vi "TestTestJunk.vi"() -> ()   [LabVIEW 2013]
uses:
  <vilib>/regexp/Match Regular Expression.xnode
panel:
  out "String":string
  out "VP/F1 5":bool
  out "VP/F1":bool
  out "VP/F1 2":bool
  out "VP/F1 4":bool
  out "VP/F1 3":bool
  out "Pass/Fail1 2":bool
  out "Pass/Fail1":bool
  out "Pass/Fail1 4":bool
  out "Pass/Fail1 3":bool
  out "Pass/Fail1 5":bool
  out "Percent 1":dbl
  out "Percent 2":dbl
  out "Voltage 1":dbl
  out "Percent 3":dbl
  out "Percent 4":dbl
  out "Voltage 2":dbl
  out "Voltage 4":dbl
  out "Voltage 3":dbl
  out "Percent 5":dbl
  out "Voltage 5":dbl
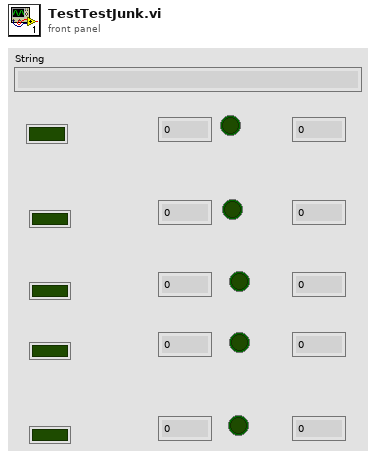
[diagram p1: front panel]
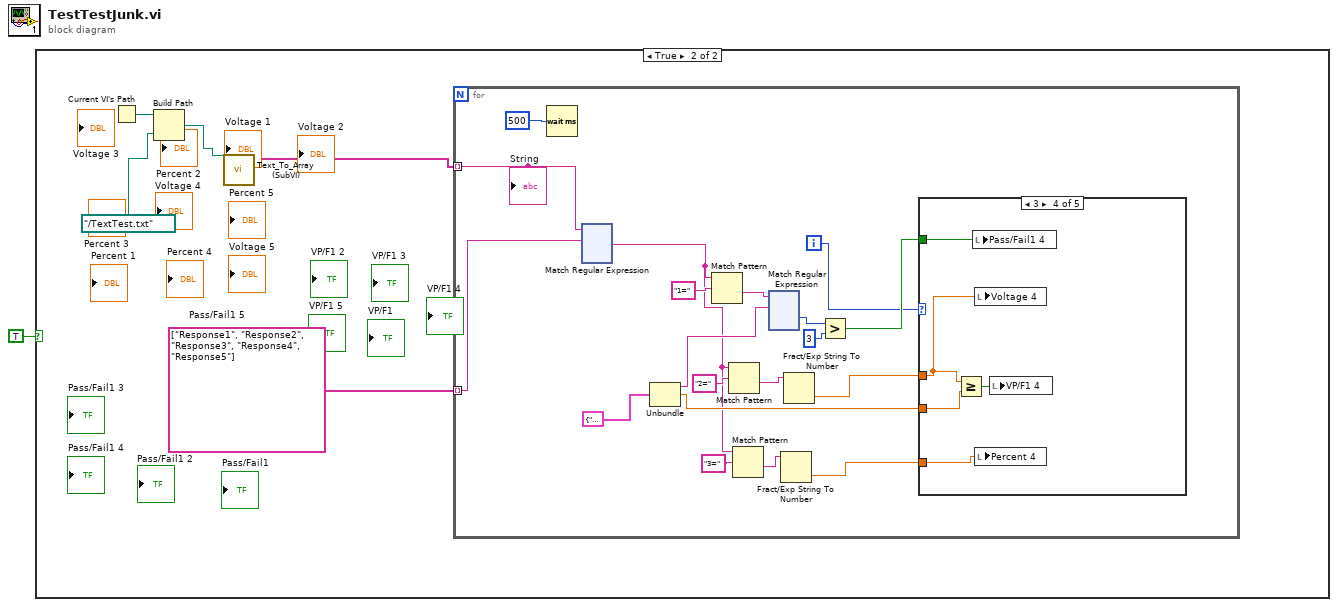
[diagram p0: block diagram]
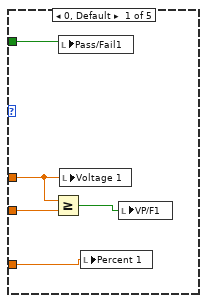
[diagram p3: hidden frame]
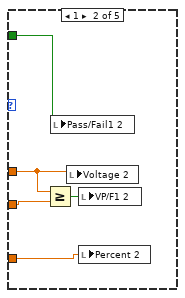
[diagram p4: hidden frame]
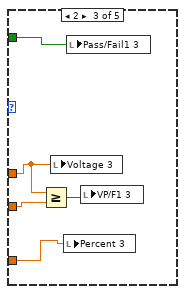
[diagram p5: hidden frame]
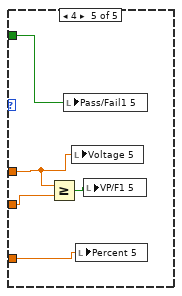
[diagram p6: hidden frame]
diagram:
  n1 = case shown="True" TRUE {
    frame False {
    }
    frame True {
      n2 = Current VI's Path() -> (path=w4:path)
      n3 = Build Path(base path=w4, name or relative path=path "../TextTest.txt") -> (appended path=w2:path)
      n4 = call "Text_To_Array (SubVI).vi"("Path"=w2) -> ("Array"=w5:string[])  [unwired: 8 in, 2 out]
      n5 = for {
        tunnel: w5 -> [w14] mode=indexing
        tunnel: string[] ["Response1", "Response2", "Response3", "Response4", "Response5"] -> [w13] mode=indexing
        i -> [w12]
        n6 = Wait (ms)(milliseconds to wait=500) -> ()  [unwired: 1 out]
        n7 = xnode "Match Regular Expression"("input string"=w14, "regular expression"=w13) -> ("after match"=w9:string)  [unwired: 4 in, 4 out]
        n8 = Unbundle(cluster{string, dbl, i32} {"PASS", 3.3, 80}) -> (w24:string, w11:dbl)  [unwired: 1 out]
        n9 = Match Pattern(string=w9, regular expression="1=") -> (after substring=w21:string)  [unwired: 1 in, 3 out]
        n10 = Match Pattern(string=w9, regular expression="2=") -> (after substring=w16:string)  [unwired: 1 in, 3 out]
        n11 = Match Pattern(string=w9, regular expression="3=") -> (after substring=w8:string)  [unwired: 1 in, 3 out]
        n12 = xnode "Match Regular Expression"("input string"=w21, "regular expression"=w24) -> ("offset past match"=w20:i32)  [unwired: 4 in, 4 out]
        n13 = Fract/Exp String To Number(string=w8) -> (number=w7:dbl)  [unwired: 3 in, 1 out]
        n14 = Fract/Exp String To Number(string=w16) -> (number=w15:dbl)  [unwired: 3 in, 1 out]
        n15 = Greater?(x=w20, y=3) -> (0:w18:bool)
        n16 = case shown="3" w12 {
          tunnel: w18 -> [w30 w35 w40 w45 w50]
          tunnel: w15 -> [w29 w34 w39 w44 w49]
          tunnel: w11 -> [w28 w33 w38 w43 w48]
          tunnel: w7 -> [w26 w31 w36 w41 w46]
          frame 0, Default {
            n17 = Greater Or Equal?(x=w29, y=w28) -> (x >= y?=w27:bool)
            n18 = local write "Pass/Fail1"(w30) -> ()
            n19 = local write "Voltage 1"(w29) -> ()
            n20 = local write "Percent 1"(w26) -> ()
            n21 = local write "VP/F1"(w27) -> ()
          }
          frame 1 {
            n22 = Greater Or Equal?(x=w34, y=w33) -> (x >= y?=w32:bool)
            n23 = local write "Pass/Fail1 2"(w35) -> ()
            n24 = local write "Voltage 2"(w34) -> ()
            n25 = local write "VP/F1 2"(w32) -> ()
            n26 = local write "Percent 2"(w31) -> ()
          }
          frame 2 {
            n27 = Greater Or Equal?(x=w39, y=w38) -> (x >= y?=w37:bool)
            n28 = local write "Voltage 3"(w39) -> ()
            n29 = local write "Percent 3"(w36) -> ()
            n30 = local write "Pass/Fail1 3"(w40) -> ()
            n31 = local write "VP/F1 3"(w37) -> ()
          }
          frame 3 {
            n32 = Greater Or Equal?(x=w44, y=w43) -> (x >= y?=w42:bool)
            n33 = local write "Pass/Fail1 4"(w45) -> ()
            n34 = local write "Voltage 4"(w44) -> ()
            n35 = local write "Percent 4"(w41) -> ()
            n36 = local write "VP/F1 4"(w42) -> ()
          }
          frame 4 {
            n37 = Greater Or Equal?(x=w49, y=w48) -> (x >= y?=w47:bool)
            n38 = local write "Pass/Fail1 5"(w50) -> ()
            n39 = local write "Voltage 5"(w49) -> ()
            n40 = local write "Percent 5"(w46) -> ()
            n41 = local write "VP/F1 5"(w47) -> ()
          }
        }
        "String" <- w14
      }
    }
  }
